vi "test_DependencyList_FilterByMatchingString.vi"() -> (3 "Pass?":bool)   [LabVIEW 2020, in "Tests.DependencyInspection.lvlib"]
uses:
  Tests.DependencyInspection.lvlib
  CDependencyList/CDependencyList.lvclass
  ItemInfo.ctl
  CDependencyList/ListGenerationOptions.ctl
panel:
  out "Array":string[](array[string])
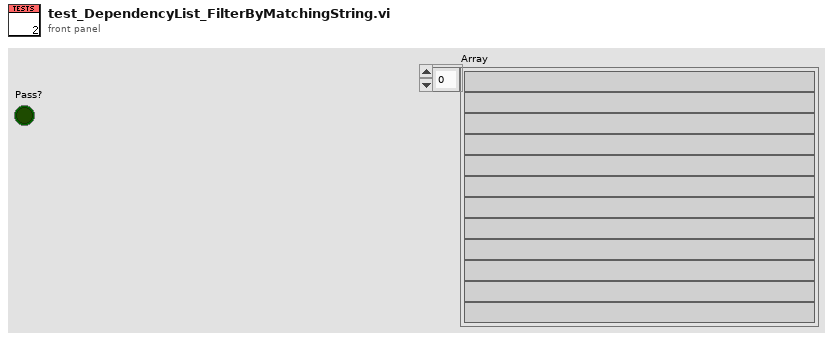
[diagram p1: front panel]
types:
  T1 = typedef "Tests.DependencyInspection.lvlib/ItemInfo.ctl" = cluster{"path":path, "delimited name":string}
  T2 = typedef "DependencyInspection.lvlib/CDependencyList.lvclass/ListGenerationOptions.ctl" = cluster{"exclude external?":bool, "exclude instances?":bool, "separate tests?":bool, "Root Path":path}
  T3 = typedef "NI_FileType.lvlib/LVFileType.ctl" = enum32{"Invalid file", "Unknown type", "Instrument", "Control", "Polymorphic VI", "Project", "Library", "LVClass", "XControl", "XNode", "Shared library", ".NET assembly", "ActiveX interface", "CIN", "Run-time menu", "Palette menu", "Help file", "LLB", "XNode Edit Dependency", "Class Private Data Control", "Statechart", "MathScript .m file", "Ladder Diagram", "LVLibp", "XNode Build Dependency"}
  T4 = cluster{"path":path, "delimited name":string, "type":T3, "iState":u32, "iStyle":u16, "wStyle":u16, "buttons":u16, "viflags":u32, "viflags2":u32, "links":u32[]}[]
  T5 = typedef "DependencyInspection.lvlib/CDependencyList.lvclass/DependencyList.ctl" = map{string, refnum<class "ILabVIEWItem.lvclass">}
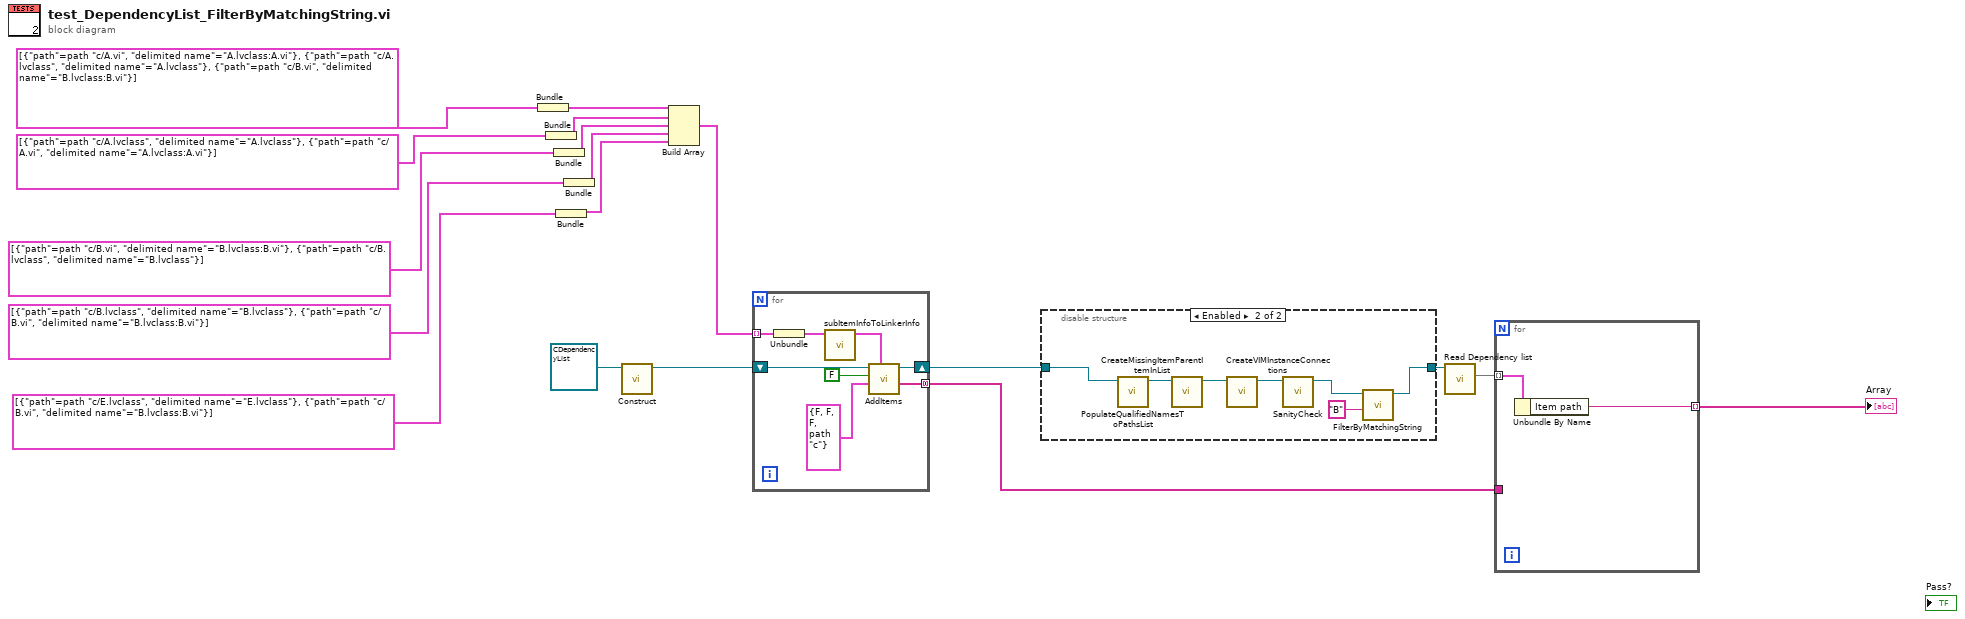
[diagram p0: block diagram]
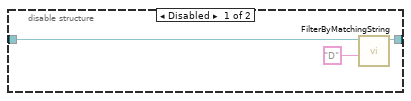
[diagram p2: hidden frame]
diagram:
  n1 = Bundle(T1[] [{"path"=path "c:/A.vi", "delimited name"="A.lvclass:A.vi"}, {"path"=path "c:/A.lvclass", "delimited name"="A.lvclass"}, {"path"=path "c:/B.vi", "delimited name"="B.lvclass:B.vi"}]) -> (w7:cluster{T1[]})  [unwired: 1 in]
  n2 = Bundle(T1[] [{"path"=path "c:/A.lvclass", "delimited name"="A.lvclass"}, {"path"=path "c:/A.vi", "delimited name"="A.lvclass:A.vi"}]) -> (w6:cluster{T1[]})  [unwired: 1 in]
  n3 = Bundle(T1[] [{"path"=path "c:/B.vi", "delimited name"="B.lvclass:B.vi"}, {"path"=path "c:/B.lvclass", "delimited name"="B.lvclass"}]) -> (w5:cluster{T1[]})  [unwired: 1 in]
  n4 = Bundle(T1[] [{"path"=path "c:/E.lvclass", "delimited name"="E.lvclass"}, {"path"=path "c:/B.vi", "delimited name"="B.lvclass:B.vi"}]) -> (w1:cluster{T1[]})  [unwired: 1 in]
  n5 = Bundle(T1[] [{"path"=path "c:/B.lvclass", "delimited name"="B.lvclass"}, {"path"=path "c:/B.vi", "delimited name"="B.lvclass:B.vi"}]) -> (w4:cluster{T1[]})  [unwired: 1 in]
  n6 = call-dynamic "Construct.vi"("CDependencyList in"=refnum<class "CDependencyList.lvclass"> refnum) -> ("CDependencyList out"=w17:refnum<class "CDependencyList.lvclass">)  [unwired: 9 in, 1 out]
  n7 = Build Array(w7, w6, w5, w4, w1) -> (w3:cluster{T1[]}[])
  n8 = for {
    tunnel: [w21] -> w12 mode=concatenating
    shift-right: [w25] -> w16
    shift-left: w17 -> [w26]
    tunnel: w3 -> [w20] mode=indexing
    n9 = Unbundle(w20) -> (w19:T1[])
    n10 = call "subItemInfoToLinkerInfo.vi"("Item info[]"=w19) -> ("Linker.Read Info From File"=w24:T4)  [unwired: 10 in]
    n11 = call-dynamic "AddItems.vi"("Linker.Read Info From File"=w24, "Settings"=T2 {"exclude external?"=FALSE, "exclude instances?"=FALSE, "separate tests?"=FALSE, "Root Path"=path "c:/"}, "Shallow deps?"=FALSE, "CDependencyList in"=w26) -> ("Debug messages"=w21:string[], "CDependencyList out"=w25:refnum<class "CDependencyList.lvclass">)  [unwired: 4 in, 2 out]
  }
  n12 = disable-structure shown="Enabled" {
    disable-tunnel: w16 -> [w27 w33]
    disable-tunnel: [w28 w31] -> w15
    frame Disabled {
      n13 = call-dynamic "FilterByMatchingString.vi"("Target filter"="D", "CDependencyList in"=w27) -> ("CDependencyList out"=w28:refnum<class "CDependencyList.lvclass">)  [unwired: 8 in, 1 out]
    }
    frame Enabled {
      n14 = call-dynamic "PopulateQualifiedNamesToPathsList.vi"("CDependencyList in"=w33) -> ("CDependencyList out"=w34:refnum<class "CDependencyList.lvclass">)  [unwired: 9 in, 1 out]
      n15 = call-dynamic "CreateMissingItemParentItemInList.vi"("CDependencyList in"=w34) -> ("CDependencyList out"=w36:refnum<class "CDependencyList.lvclass">)  [unwired: 9 in, 1 out]
      n16 = call-dynamic "CreateVIMInstanceConnections.vi"("CDependencyList in"=w36) -> ("CDependencyList out"=w35:refnum<class "CDependencyList.lvclass">)  [unwired: 9 in, 1 out]
      n17 = call-dynamic "SanityCheck.vi"("CDependencyList in"=w35) -> ("CDependencyList out"=w32:refnum<class "CDependencyList.lvclass">)  [unwired: 8 in, 2 out]
      n18 = call-dynamic "FilterByMatchingString.vi"("Target filter"="B", "CDependencyList in"=w32) -> ("CDependencyList out"=w31:refnum<class "CDependencyList.lvclass">)  [unwired: 8 in, 1 out]
    }
  }
  n19 = call-dynamic "Read Dependency list.vi"("CDependencyList in"=w15) -> ("Dependency List"=w14:T5)  [unwired: 9 in, 1 out]
  n20 = for {
    tunnel: w14 -> [w38] mode=indexing
    tunnel: [w37] -> w13 mode=indexing
    tunnel: w12 -> [_]
    n21 = Unbundle By Name(w38) -> ("Item path"=w37:string)
  }
  "Array" <- w13
